vi "836_CameraGet Image From TCP.vi"(7 "Camera Mode":u16(ring) items=["Camera Off", "USB Camera SW", "USB Camera HW", "IP Camera"], 8 "error in (no error)":errorcluster, 9 "USB":bool, 10 "Image In":T1, 11 "connection ID":refnum<k5>) -> (0 "error out":errorcluster, 1 "Size":i32, 2 "Image Out":T1, 3 "connection ID (dup)":refnum<k5>)   [LabVIEW 2015]
doc: "This software is licensed. Open the labview\\readme\\WPI Robotics Library Open Source License.txt file for more information."
uses:
  <vilib>/vision/Image Controls.llb/IMAQ Image.ctl
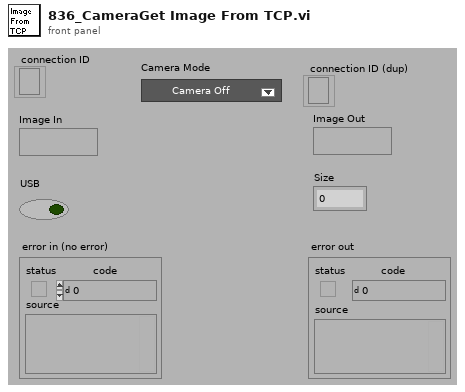
[diagram p1: front panel]
types:
  T1 = typedef "IMAQ Image.ctl" = refnum<image>
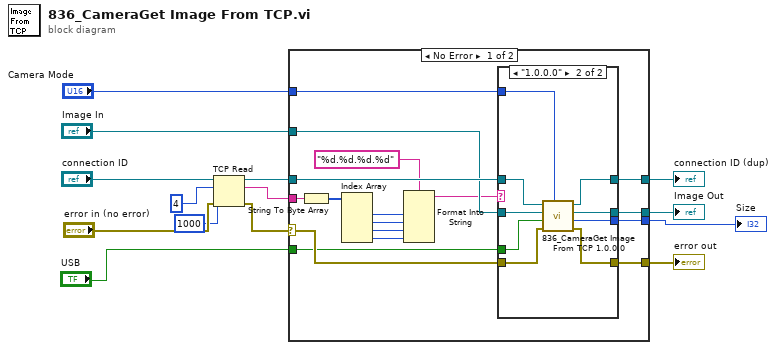
[diagram p0: block diagram]
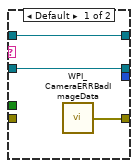
[diagram p2: hidden frame]
diagram:
  n1 = TCP Read(connection ID="connection ID", bytes to read=4, error in (no error)="error in (no error)", 9:1000 ("timeout ms (25000)")) -> (connection ID out=w14:refnum<k5>, data out=w10:string, error out=w5:errorcluster)  [unwired: 1 out]
  n2 = case shown="No Error" w5 {
    selector: w5 -> [w18 w44]
    tunnel: w14 -> [w31 w46]
    tunnel: "Image In" -> [w30 w45]
    tunnel: w10 -> [w23 _]
    tunnel: [w21 w44] -> w8
    tunnel: [w20 w45] -> w7
    tunnel: [w19 w46] -> w6
    tunnel: "USB" -> [w17 _]
    tunnel: [w16 _] -> w3
    tunnel: "Camera Mode" -> [w15 _]
    frame No Error {
      n3 = String To Byte Array(string=w23) -> (unsigned byte array=w24:u8[])
      n4 = Index Array(array=w24) -> (element #1=w26:u8, element #2=w27:u8, element #3=w28:u8, element #4=w29:u8)  [unwired: 4 in]
      n5 = Format Into String(format string="%d.%d.%d.%d", w26, w27, w28, w29) -> (resulting string=w22:string)  [unwired: 2 in, 1 out]
      n6 = case shown="\"1.0.0.0\"" w22 {
        tunnel: w31 -> [w34 w43]
        tunnel: w30 -> [w33 w42]
        tunnel: w18 -> [_ w41]
        tunnel: [w32 w40] -> w21
        tunnel: [w33 w39] -> w20
        tunnel: [w34 w38] -> w19
        tunnel: w17 -> [_ w37]
        tunnel: [_ w36] -> w16
        tunnel: w15 -> [_ w35]
        frame Default {
          n7 = call <vilib>:"WPI_CameraERRBadImageData.vi"() -> ("error out"=w32:errorcluster)
        }
        frame "1.0.0.0" {
          n8 = call "836_CameraGet Image From TCP 1.0.0.0.vi"("Camera Mode"=w35, "error in (no error)"=w41, "USB"=w37, "Image In"=w42, "connection ID"=w43) -> ("error out"=w40:errorcluster, "Size"=w36:i32, "Image Out"=w39:T1, "connection ID out"=w38:refnum<k5>)  [unwired: 1 in, 2 out]
        }
      }
    }
    frame Error {
    }
  }
  "error out" <- w8
  "Image Out" <- w7
  "connection ID (dup)" <- w6
  "Size" <- w3
